vi "Handle Water Cooling Station.vi"(0 "reference in":refnum<class "PM_Group.lvclass">, 11 "error in (no error)":errorcluster) -> (4 "reference out":refnum<class "PM_Group.lvclass">, 15 "error out":errorcluster)   [LabVIEW 2019, in "PM_Group.lvclass"]
uses:
  PM_Group.lvclass
  PM_Group.lvclass/PM_Group.ctl
  FPGA/TypeDef/AI index.ctl
  AI_class/AI.lvclass/AI.ctl
  AnalogComparator_class/AnalogComparator.lvclass/AnalogComparator.ctl
  FPGA/TypeDef/DO index.ctl
  AnalogComparator_class/GetStatus.vi
  AI_class/AI.lvclass
  FPGA_API_class/FPGA API.lvclass
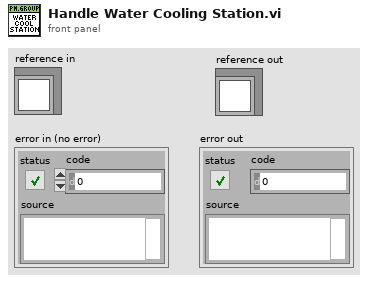
[diagram p1: front panel]
types:
  T1 = typedef "AI index.ctl" = u8
  T2 = typedef "DO index.ctl" = u8
  T3 = typedef "AI_Data.ctl" = cluster{"Stat Data":T4, "OutOfRangeMax":bool, "OutOfRangeMin":bool, "HIHI":bool, "HI":bool, "LO":bool, "LOLO":bool}
  T4 = typedef "AI Statistics Data.ctl" = cluster{"raw mean":dbl, "scl mean":dbl, "raw mean 1Hz":dbl, "scl mean 1Hz":dbl, "raw standard deviation":dbl, "raw max value":dbl, "raw min value":dbl}
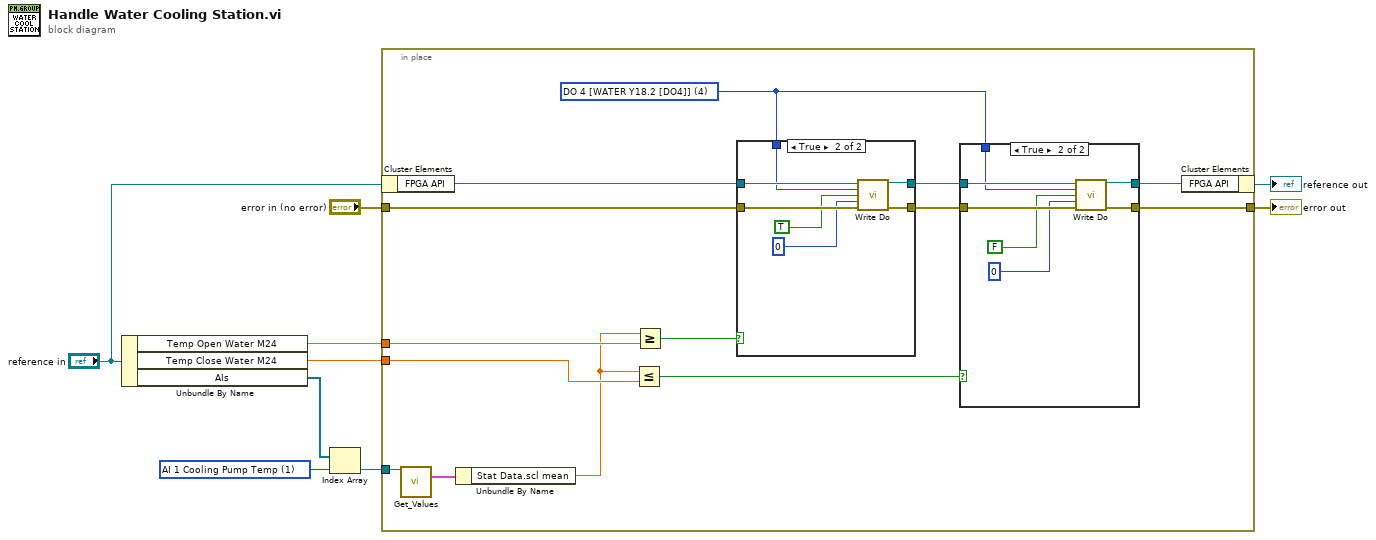
[diagram p0: block diagram]
diagram:
  w6 = T1 1 items=["AI 0 Cooling Pump Level", "AI 1 Cooling Pump Temp", "AI 2 Oil Supply Level", "AI 3 Oil Supply Temp", "AI 4 ", "AI 5 Pressure Haskel", "AI 6 Pressure DUT", "AI 7 Pressure Chamber", "AI 8 Pressure Air inlet", "AI 9 Pressure Air outlet", "AI 10 Pressure Messure Line"] ("AI index")
  n1 = Unbundle By Name("reference in") -> ("Temp Open Water M24"=w3:dbl, "Temp Close Water M24"=w4:dbl, "AIs"=w5:refnum<class "AI.lvclass">[])
  n2 = Index Array(array=w5, index=w6) -> (element=w7:refnum<class "AI.lvclass">)
  n3 = in-place {
    in-place-border: w3 -> [w13]
    in-place-border: w4 -> [w14]
    in-place-border: w7 -> [w23]
    in-place-border: "error in (no error)" -> [w21]
    in-place-border: [w16] -> w9
    w10 = T2 4 items=["DO 0 [KP1 [DO 0]]", "DO 1 [ON KP2 [DO 1]]", "DO 2 [ON KP3 [DO 2]]", "DO 3 [WATER Y18.1 [DO3]]", "DO 4 [WATER Y18.2 [DO4]]", "DO 5 [KP6 Y29.1 33.7]", "DO 6 [KP7 Y29.2 33.8]", "DO 7 [KP8 Y29.3 33.9]", "DO 8 [KP9 Y29.4  33.12]", "DO 9 [KP10 Y29.5 33.1]", "DO 10 [KP11 Y29.6 33.2]", "DO 11 [KP12 Y29.7  33.13]", "DO 12 [KP13 Y29.8  33.11]", "DO 13 [KP14 Y29.9 33.10]", "DO 14 [KP15 Y29.10  33.6]", "DO 15 [KP16 Y29.11  33.5]", "DO 16 [KP17 Y29.12  33.4]", "DO 17 [KP18 Y29.13 33.3]", "DO 18 [AIR KP19]", "DO 19 [STEP DRIVE EN KP20]", "DO 20 [KP21 Y44.1 OPEN]", "DO 21 [ KP22 Y44.1 CLOSE]", "DO 22 [ KP23 Y44.2 OPEN]", "DO 23", "DO 24 [STEP DRIVE 1]", "DO 25 [STEP DRIVE 2]"] ("#DO")
    n4 = in-place-cluster #1("reference in") -> ("FPGA API"=w20:refnum<class "FPGA API.lvclass">)
    n5 = call "Get_Values.vi"("reference in"=w23) -> ("Data"=w22:T3)  [unwired: 14 in]
    n6 = Unbundle By Name(w22) -> ("Stat Data.scl mean"=w11:dbl)
    n7 = Less Or Equal?(x=w11, y=w14) -> (x <= y?=w12:bool)
    n8 = Greater Or Equal?(x=w11, y=w13) -> (x >= y?=w19:bool)
    n9 = case shown="True" w19 {
      tunnel: w21 -> [w33 w39]
      tunnel: w20 -> [w34 w41]
      tunnel: [w34 w40] -> w15
      tunnel: [w33 w38] -> w17
      tunnel: w10 -> [_ w36]
      frame False {
      }
      frame True {
        n10 = call "Write Do.vi"("FPGA API in"=w41, "#DO"=w36, "value"=TRUE, "Time uSec"=u32 0, "error in (no error)"=w39) -> ("FPGA API out"=w40:refnum<class "FPGA API.lvclass">, "error out"=w38:errorcluster)  [unwired: 9 in]
      }
    }
    n11 = case shown="True" w12 {
      tunnel: w15 -> [w24 w32]
      tunnel: [w24 w29] -> w18
      tunnel: w17 -> [w25 w31]
      tunnel: [w25 w30] -> w16
      tunnel: w10 -> [_ w28]
      frame False {
      }
      frame True {
        n12 = call "Write Do.vi"("FPGA API in"=w32, "#DO"=w28, "value"=FALSE, "Time uSec"=u32 0, "error in (no error)"=w31) -> ("FPGA API out"=w29:refnum<class "FPGA API.lvclass">, "error out"=w30:errorcluster)  [unwired: 9 in]
      }
    }
    n13 = in-place-cluster #1("FPGA API"=w18) -> (→"reference out":refnum<class "PM_Group.lvclass">)
  }
  "error out" <- w9
